vi "CASCADE ILLUMINATION LED VALIDATION_PATTERN_MATCH - Copy.vi"(0 "Template File Path (Pattern Locate Datum)":path=path "C:/mtp/Site_Ne_sch/Test_Templates/IMAGES/XD_ILLUMINATION_LED.png", 1 "Test File Path":path=path "C:/TEST_DATA/ILLUMINATION/19085010550261_0_13_49_ILLUMINATION_1.bmp", 7 "error in":errorcluster) -> (20 "Matches (Pattern Locate Datum)":T3(array[cluster])=[{"Position"={"x"=681.0, "y"=270.0}, "Angle"=0.0, "Scale"=1.0, "Score"=999.99994, "Bounding Box"=[{"x"=490.0, "y"=178.0}, {"x"=872.0, "y"=178.0}, {"x"=872.0, "y"=362.0}, {"x"=490.0, "y"=362.0}, {"x"=490.0, "y"=178.0}]}] {"Bounding Box"."y" format="%.2f"; "Bounding Box"."x" format="%.2f"; "Position"."y" format="%.2f"; "Position"."x" format="%.2f"; "Score" format="%.2f"; "Scale" format="%.2f"; "Angle" format="%.2f"}, 21 "Calibrated Matches (Pattern Locate Datum)":T3(array[cluster])=[{"Position"={"x"=681.0, "y"=270.0}, "Angle"=0.0, "Scale"=1.0, "Score"=999.99994, "Bounding Box"=[{"x"=490.0, "y"=178.0}, {"x"=872.0, "y"=178.0}, {"x"=872.0, "y"=362.0}, {"x"=490.0, "y"=362.0}, {"x"=490.0, "y"=178.0}]}] {"Bounding Box"."y" format="%.2f"; "Bounding Box"."x" format="%.2f"; "Position"."y" format="%.2f"; "Position"."x" format="%.2f"; "Score" format="%.2f"; "Scale" format="%.2f"; "Angle" format="%.2f"}, 22 "Number of Matches (Pattern Locate Datum)":i32=1, 23 "Coordinate System Out (Set Coordinate Right Datum)":T2={"Reference System"={"Origin"={"X"=1298.5, "Y"=413.5}, "Angle (deg)"=0.0, "Axis Reference"=0}, "Measurement System"={"Origin"={"X"=681.0, "Y"=270.0}, "Angle (deg)"=0.0, "Axis Reference"=0}} {"Measurement System"."Axis Reference" items=["Direct", "Indirect"]; "Measurement System"."Angle (deg)" format="%.2f"; "Measurement System"."Origin"."Y" format="%.2f"; "Measurement System"."Origin"."X" format="%.2f"; "Reference System"."Axis Reference" items=["Direct", "Indirect"]; "Reference System"."Angle (deg)" format="%.2f"; "Reference System"."Origin"."Y" format="%.2f"; "Reference System"."Origin"."X" format="%.2f"}, 24 "Matches (real-world)[0].Score":sgl=999.99994, 27 "error out":errorcluster)   [LabVIEW 2014]
uses:
  <vilib>/vision/NI_Vision_Development_Module.lvlib
panel:
  out "Image Out":T1(plugin-control)
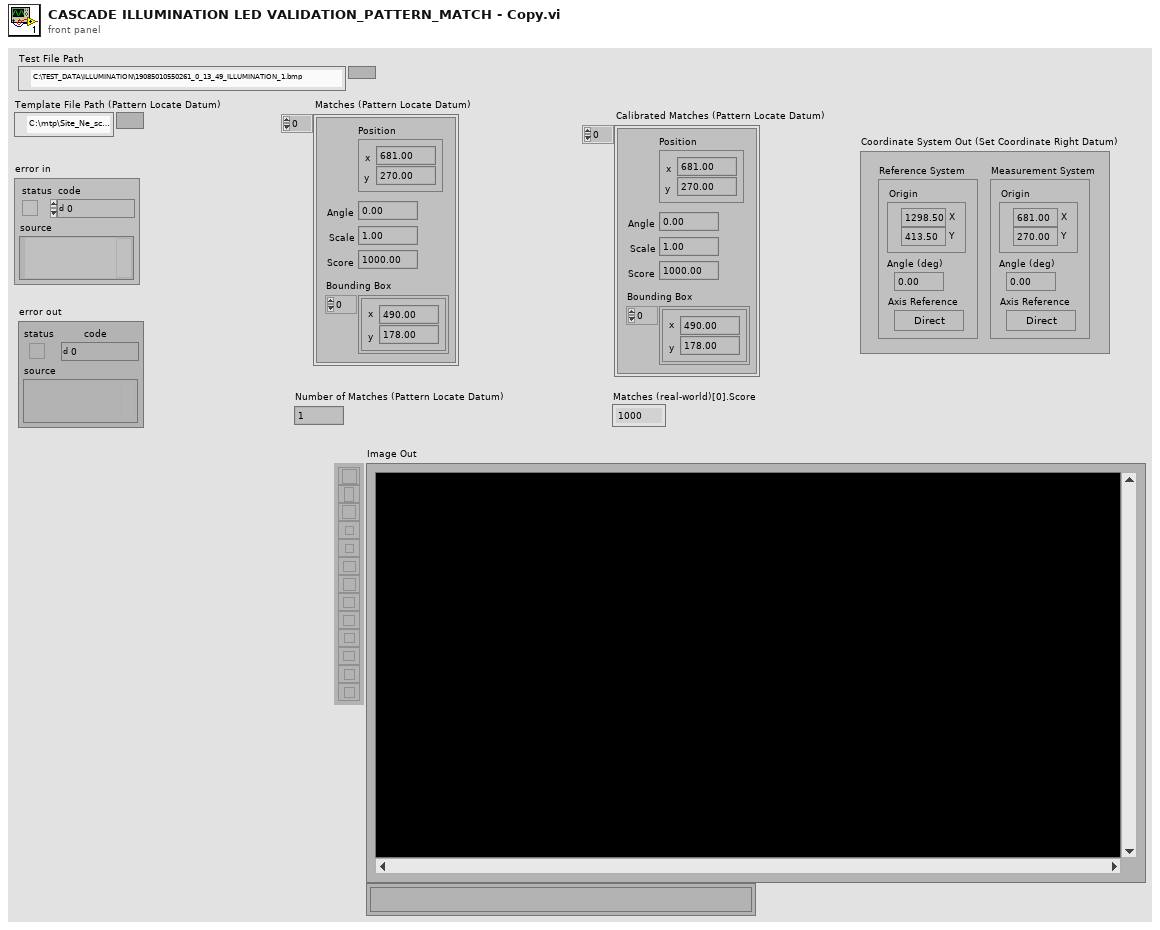
[diagram p1: front panel]
types:
  T1 = typedef "IMAQ Image.ctl" = refnum<image>
  T2 = cluster{"Reference System":cluster{"Origin":cluster{"X":sgl, "Y":sgl}, "Angle (deg)":sgl, "Axis Reference":u32}, "Measurement System":cluster{"Origin":cluster{"X":sgl, "Y":sgl}, "Angle (deg)":sgl, "Axis Reference":u32}}
  T3 = cluster{"Position":cluster{"x":sgl, "y":sgl}, "Angle":sgl, "Scale":sgl, "Score":sgl, "Bounding Box":cluster{"x":sgl, "y":sgl}[]}[]
  T4 = enum16{"Reset", "Update Coordinate System", "Get Coordinate System"}
  T5 = enum16{"Horizontal Motion", "Vertical Motion", "Horizontal and Vertical Motion", "Horizontal, Vertical and Angular Motion"}
  T6 = cluster{"Origin":cluster{"X":sgl, "Y":sgl}, "Angle (deg)":sgl, "Axis Reference":u32}
  T7 = cluster{"Number of Matches Requested":i32, "Minimum Match Score":sgl, "Angle Ranges":cluster{"Start Angle":sgl, "End Angle":sgl}[]}
  T8 = cluster{"Global Rectangle":i32[], "Contours":cluster{"ID":enum32{"External", "Internal"}, "Type":u32, "Coordinates":i32[]}[]}
  T9 = typedef "Image Type" = u32
  T10 = cluster{"Matches (real-world)[0]":cluster{"Position":cluster{"x":sgl, "y":sgl}, "Angle":sgl, "Scale":sgl, "Score":sgl, "Bounding Box":cluster{"x":sgl, "y":sgl}[]}, "Matches (real-world)[1]":cluster{"Position":cluster{"x":sgl, "y":sgl}, "Angle":sgl, "Scale":sgl, "Score":sgl, "Bounding Box":cluster{"x":sgl, "y":sgl}[]}, "Matches (real-world)[2]":cluster{"Position":cluster{"x":sgl, "y":sgl}, "Angle":sgl, "Scale":sgl, "Score":sgl, "Bounding Box":cluster{"x":sgl, "y":sgl}[]}, "Matches (real-world)[3]":cluster{"Position":cluster{"x":sgl, "y":sgl}, "Angle":sgl, "Scale":sgl, "Score":sgl, "Bounding Box":cluster{"x":sgl, "y":sgl}[]}, "Matches (real-world)[4]":cluster{"Position":cluster{"x":sgl, "y":sgl}, "Angle":sgl, "Scale":sgl, "Score":sgl, "Bounding Box":cluster{"x":sgl, "y":sgl}[]}, "Matches (real-world)[5]":cluster{"Position":cluster{"x":sgl, "y":sgl}, "Angle":sgl, "Scale":sgl, "Score":sgl, "Bounding Box":cluster{"x":sgl, "y":sgl}[]}, "Matches (real-world)[6]":cluster{"Position":cluster{"x":sgl, "y":sgl}, "Angle":sgl, "Scale":sgl, "Score":sgl, "Bounding Box":cluster{"x":sgl, "y":sgl}[]}, "Matches (real-world)[7]":cluster{"Position":cluster{"x":sgl, "y":sgl}, "Angle":sgl, "Scale":sgl, "Score":sgl, "Bounding Box":cluster{"x":sgl, "y":sgl}[]}, "Matches (real-world)[8]":cluster{"Position":cluster{"x":sgl, "y":sgl}, "Angle":sgl, "Scale":sgl, "Score":sgl, "Bounding Box":cluster{"x":sgl, "y":sgl}[]}}
  T11 = typedef "IMAQ Coordinate System" = cluster{"Reference System":cluster{"Origin":cluster{"X":sgl, "Y":sgl}, "Angle (deg)":sgl, "Axis Reference":u32}, "Measurement System":cluster{"Origin":cluster{"X":sgl, "Y":sgl}, "Angle (deg)":sgl, "Axis Reference":u32}}
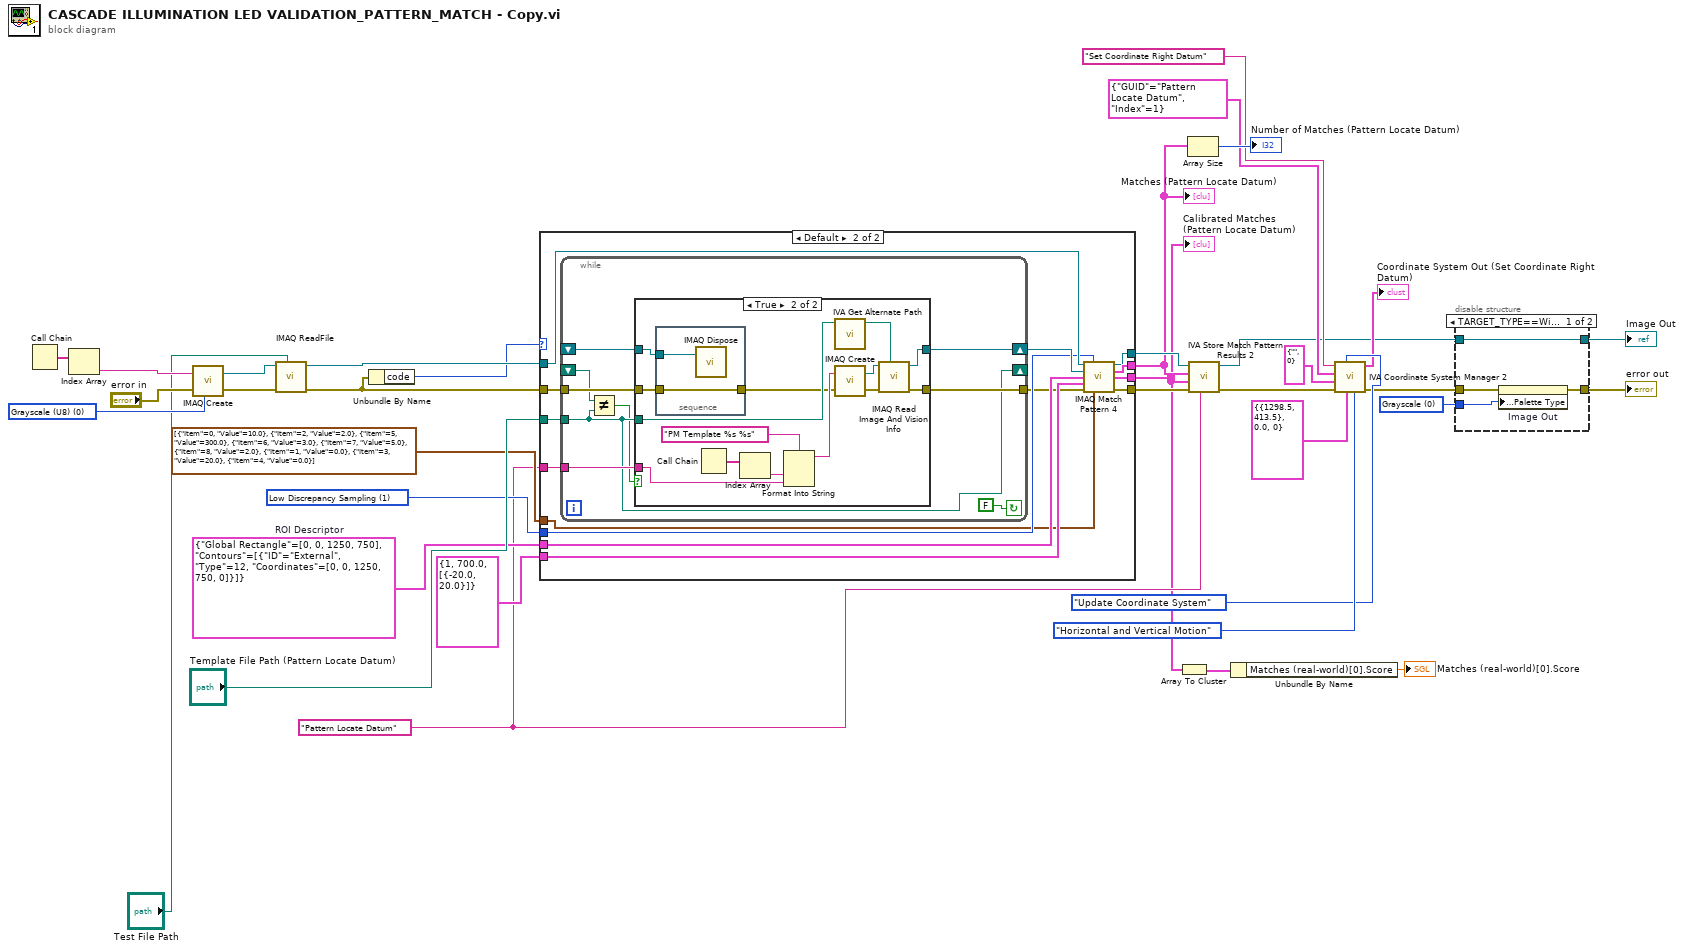
[diagram p0: block diagram]
diagram:
  w5 = u32 0 items=["Grayscale", "Binary", "Gradient", "Rainbow", "Temperature", "User Defined"] ("Palette")
  w24 = 1 items=["All", "Low Discrepancy Sampling", "Grayscale Value Pyramid", "Gradients Pyramid"] ("Algorithm")
  w19 = "Pattern Locate Datum" ("Step Name")
  w23 = T8 {"Global Rectangle"=[0, 0, 1250, 750], "Contours"=[{"ID"=enum."External", "Type"=12, "Coordinates"=[0, 0, 1250, 750, 0]}]}  # ROI Descriptor
  w31 = T9 0 items=["Grayscale (U8)", "Grayscale (I16)", "Grayscale (SGL)", "Complex (CSG)", "RGB (U32)", "HSL (U32)", "RGB (U64)", "Grayscale (U16)"] ("Image Type")
  n1 = Call Chain() -> (call chain=w33:string[])
  n2 = Index Array(array=w33) -> (element=w32:string)  [unwired: 1 in]
  n3 = call "IMAQ Create"("Image Name"=w32, "Image Type"=w31, "error in (no error)"="error in") -> ("New Image"=w36:T1, "error out"=w35:errorcluster)  [unwired: 1 in, 1 out]
  n4 = call "IMAQ ReadFile"("File Path"="Test File Path", "error in (no error)"=w35, "Image"=w36) -> ("error out"=w26:errorcluster, "Image Out"=w29:T1)  [unwired: 2 in, 5 out]
  n5 = Unbundle By Name(w26) -> ("code"=w25:i32)
  n6 = case shown="Default" w25 {
    tunnel: "Template File Path (Pattern Locate Datum)" -> [_ w51]
    tunnel: w26 -> [_ w50]
    tunnel: w29 -> [w37 w45]
    tunnel: [_ w46] -> w28
    tunnel: [_ w47] -> w18
    tunnel: [w37 w44] -> w27
    tunnel: w19 -> [_ w49]
    tunnel: w24 -> [_ w43]
    tunnel: w23 -> [_ w42]
    tunnel: T7 {"Number of Matches Requested"=1, "Minimum Match Score"=700.0, "Angle Ranges"=[{"Start Angle"=-20.0, "End Angle"=20.0}]} ("Parameters") -> [_ w41]
    tunnel: cluster{"Item":u16, "Value":dbl}[] [{"Item"=0, "Value"=10.0}, {"Item"=2, "Value"=2.0}, {"Item"=5, "Value"=300.0}, {"Item"=6, "Value"=3.0}, {"Item"=7, "Value"=5.0}, {"Item"=8, "Value"=2.0}, {"Item"=1, "Value"=0.0}, {"Item"=3, "Value"=20.0}, {"Item"=4, "Value"=0.0}] ("Advanced Options") -> [_ w39]
    tunnel: [_ w38] -> w3
    frame -1074396199, -1074396198 {
      # "Discard Coordinate System Error"
    }
    frame Default {
      n7 = while {
        shift-right: [w60] -> w48
        shift-left: _ -> [w59]
        tunnel: [w57] -> w40
        tunnel: w50 -> [w56]
        tunnel: w51 -> [w53]
        tunnel: w49 -> [w55]
        shift-right: [w53] -> _
        shift-left: _ -> [w54]
        stop <- FALSE continue-if-true
        n8 = Not Equal?(x=w54, y=w53) -> (x != y?=w52:bool)
        n9 = case shown="True" w52 {
          tunnel: [w62 w74] -> w60
          tunnel: w59 -> [w62 w65]
          tunnel: [w61 w71] -> w57
          tunnel: w56 -> [w61 w64]
          tunnel: w53 -> [_ w67]
          tunnel: w55 -> [_ w68]
          frame False {
          }
          frame True {
            n10 = stacked-sequence {
              tunnel: w65 -> [w78]
              tunnel: w64 -> [w77]
              tunnel: [w77] -> w63
              frame #0 {
                n11 = call "IMAQ Dispose"("Image"=w78) -> ()  [unwired: 2 in, 4 out]
              }
            }
            n12 = Call Chain() -> (call chain=w70:string[])
            n13 = Index Array(array=w70) -> (element=w69:string)  [unwired: 1 in]
            n14 = Format Into String(format string="PM Template %s %s" ("Image Name"), w69, w68) -> (resulting string=w76:string)  [unwired: 2 in, 1 out]
            n15 = call <vilib>:"IVA Get Alternate Path.vi"("Path In"=w67) -> ("Path Out"=w66:path)  [unwired: 10 out]
            n16 = call "IMAQ Create"("Image Name"=w76, "error in (no error)"=w63) -> ("New Image"=w73:T1, "error out"=w72:errorcluster)  [unwired: 2 in, 1 out]
            n17 = call "IMAQ Read Image And Vision Info"("File Path"=w66, "error in (no error)"=w72, "Image"=w73) -> ("error out"=w71:errorcluster, "Image Out"=w74:T1)  [unwired: 1 in, 6 out]
          }
        }
      }
      n18 = call "IMAQ Match Pattern 4"("Image"=w45, "Algorithm"=w43, "Template Image"=w48, "ROI Descriptor"=w42, "Parameters"=w41, "error in (no error)"=w40, "Advanced Options"=w39) -> ("Image (duplicate)"=w44:T1, "Matches (pixel)"=w47:T3, "Matches (real-world)"=w38:T3, "error out"=w46:errorcluster)  [unwired: 4 in, 1 out]
    }
  }
  "Matches (Pattern Locate Datum)" <- w18
  "Calibrated Matches (Pattern Locate Datum)" <- w3
  n19 = Array To Cluster(array=w3) -> (cluster=w2:T10)
  n20 = Array Size(array=w18) -> (size(s)=→"Number of Matches (Pattern Locate Datum)":i32)
  n21 = call <vilib>:"IVA Store Match Pattern Results 2.vi"("Step Name"=w19, "error in (no error)"=w28, "Matches (real-world)"=w3, "Matches (pixel)"=w18, "Image in"=w27) -> ("error out"=w11:errorcluster, "Image dup"=w7:T1)  [unwired: 1 in, 4 out]
  n22 = Unbundle By Name(w2) -> ("Matches (real-world)[0].Score"=→"Matches (real-world)[0].Score":sgl)
  n23 = call <vilib>:"IVA Coordinate System Manager 2.vi"("Mode"=T5."Horizontal and Vertical Motion", "Reference System"=T6 {"Origin"={"X"=1298.5, "Y"=413.5}, "Angle (deg)"=0.0, "Axis Reference"=0}, "Function"=T4."Update Coordinate System", "error in (no error)"=w11, "Angle ID"=cluster{"GUID":string, "Index":i32} {"GUID"="", "Index"=0}, "Origin ID"=cluster{"GUID":string, "Index":i32} {"GUID"="Pattern Locate Datum", "Index"=1}, "Coordinate System Name"="Set Coordinate Right Datum") -> ("error out"=w9:errorcluster, "Coordinate System Out"=→"Coordinate System Out (Set Coordinate Right Datum)":T11)  [unwired: 3 out]
  n24 = disable-structure "Conditional Disable Structure" shown="TARGET_TYPE==Windows" {
    disable-tunnel: w9 -> [w82 w83]
    disable-tunnel: [w81 w83] -> w8
    disable-tunnel: w7 -> [w80 w84]
    disable-tunnel: [w80 w84] -> w6
    disable-tunnel: w5 -> [w79 _]
    frame condition #0 (active) {
      n25 = property on="Image Out" class="ImageControl"(error in=w82, "Palette:Palette Type"=w79) -> (error out=w81:errorcluster)  [unwired: 1 in, 1 out]
    }
    frame condition #1 {
    }
  }
  "error out" <- w8
  "Image Out" <- w6
